vi "Register Events.vi"(0 "Display State In":T2={"WebView2 Ref"=refnum, "event callback refnum"=refnum, "Events"={"Navigation Complete Event"=refnum, "Source Changed Event"=refnum, "Document Title Changed Event"=refnum, "Status Bar Text Changed"=refnum, "Web Message Received"=refnum, "Window Close Requested"=refnum, "DOM Loaded"=refnum}, "Paths"={"Webview2 Native"=path "C:/Users/kleins/Desktop/webview2/microsoft.web.webview2.1.0.1370.28/build/native", "Edge Application"=path "", "User Data"=path ""}, "Environment Options"={"additionalBrowserArguments"="", "language"="", "targetCompatibleBrowserVersion"="", "allowSingleSignOnUsingOSPrimaryAccount"=FALSE}}, 9 "Container State":T5, 11 "error in (no error)":errorcluster) -> (4 "Display State Out":T2={"WebView2 Ref"=refnum, "event callback refnum"=refnum, "Events"={"Navigation Complete Event"=refnum, "Source Changed Event"=refnum, "Document Title Changed Event"=refnum, "Status Bar Text Changed"=refnum, "Web Message Received"=refnum, "Window Close Requested"=refnum, "DOM Loaded"=refnum}, "Paths"={"Webview2 Native"=path "C:/Users/kleins/Desktop/webview2/microsoft.web.webview2.1.0.1370.28/build/native", "Edge Application"=path "", "User Data"=path ""}, "Environment Options"={"additionalBrowserArguments"="", "language"="", "targetCompatibleBrowserVersion"="", "allowSingleSignOnUsingOSPrimaryAccount"=FALSE}}, 6 "Events":T1, 15 "error out":errorcluster)   [LabVIEW 2020, in "WebView2 Control.xctl"]
uses:
  WebView2 Control.xctl
  <vilib>/_xctls/Container State.ctl
  State.ctl
  E:/Labview/LV 2020/Libs/WebView2/LV-WebView2/Source/microsoft.web.webview2/lib/net45/Microsoft.Web.WebView2.WinForms.dll
  microsoft.web.webview2/lib/net45/Microsoft.Web.WebView2.WinForms.dll
  Events.ctl
  Paths.ctl
  Core Env Options.ctl
  _Raise Nav Complete Event.vi
  _Raise Navigation Starting Event.vi
  _Raise Source Changed Event.vi
  _Raise Document Title Changed.vi
  _Raise StatusBarTextChanged.vi
  _Raise WebMessageReceived.vi
  _Raise WindowCloseRequested.vi
  _Raise Dom Content Loaded.vi
  E:/Labview/LV 2020/Libs/WebView2/LV-WebView2/Source/microsoft.web.webview2/lib/net45/Microsoft.Web.WebView2.Core.dll
  microsoft.web.webview2/lib/net45/Microsoft.Web.WebView2.Core.dll
  <vilib>/_xctls/XControlSupport.lvlib
panel:
  # "Add Controls & Indicators that form the parameters of the method here. Hook them to the connector pane. Do not delete the controls & indicators that are already hooked to the connector pane.\n \nTo setup the parameters  for this method, right click on this item in the Project Tree & select \"Configure Method...\"."
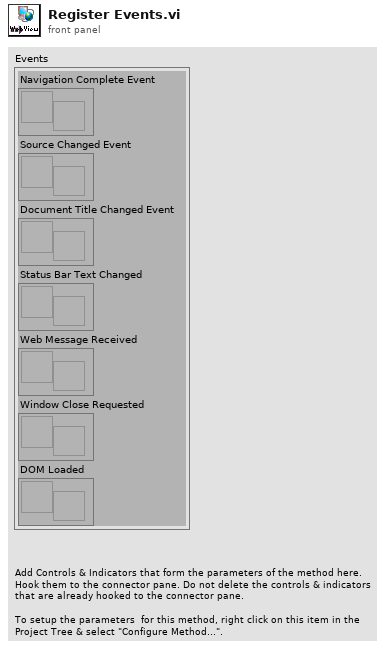
[diagram p1: front panel]
types:
  T1 = typedef "WebView2 Control.xctl/Events.ctl" = cluster{"Navigation Complete Event":refnum<user-event>, "Source Changed Event":refnum<user-event>, "Document Title Changed Event":refnum<user-event>, "Status Bar Text Changed":refnum<user-event>, "Web Message Received":refnum<user-event>, "Window Close Requested":refnum<user-event>, "DOM Loaded":refnum<user-event>}
  T2 = typedef "WebView2 Control.xctl/State.ctl" = cluster{"WebView2 Ref":refnum<data-value>, "event callback refnum":refnum<k27>, "Events":T1, "Paths":T3, "Environment Options":T4}
  T3 = typedef "WebView2 Control.xctl/Paths.ctl" = cluster{"Webview2 Native":path, "Edge Application":path, "User Data":path}
  T4 = typedef "WebView2 Control.xctl/Core Env Options.ctl" = cluster{"additionalBrowserArguments":string, "language":string, "targetCompatibleBrowserVersion":string, "allowSingleSignOnUsingOSPrimaryAccount":bool}
  T5 = typedef "XControlSupport.lvlib/Container State.ctl" = cluster{"Indicator?":bool, "Run Mode?":bool, " Refnum":refnum<vi>}
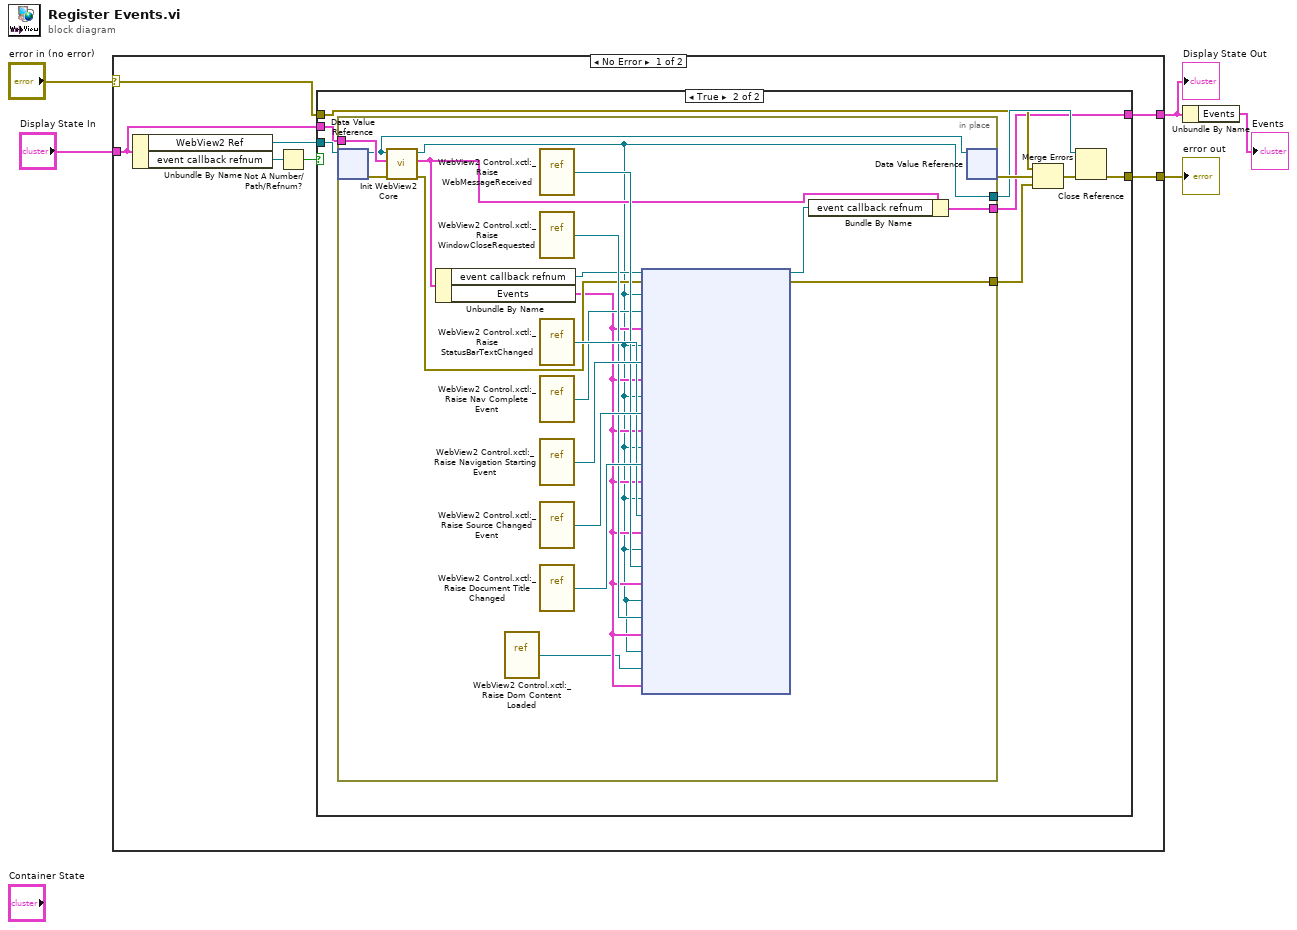
[diagram p0: block diagram]
diagram:
  n1 = case shown="No Error" "error in (no error)" {
    selector: "error in (no error)" -> [w9 w44]
    tunnel: [w8 w43] -> w2
    tunnel: "Display State In" -> [w11 w43]
    tunnel: [w10 w44] -> w4
    frame No Error {
      n2 = Unbundle By Name(w11) -> ("WebView2 Ref"=w12:refnum<data-value>, "event callback refnum"=w7:refnum<k27>)
      n3 = Not A Number/Path/Refnum?(number/path/refnum=w7) -> (NaN/Path/Refnum?=w6:bool)
      n4 = case shown="True" w6 {
        tunnel: w12 -> [_ w23]
        tunnel: w11 -> [w14 w22]
        tunnel: [w13 w21] -> w10
        tunnel: w9 -> [w13 w16]
        tunnel: [w14 w15] -> w8
        frame False {
        }
        frame True {
          n5 = in-place {
            in-place-border: [w42] -> w19
            in-place-border: [w24] -> w17
            in-place-border: w22 -> [w33]
            in-place-border: [w27] -> w15
            n6 = in-place-dvr #1(w23) -> (w32:refnum<k24>, w31:errorcluster)
            n7 = call "Init WebView2 Core.vi"("error in (no error)"=w31, "Display State In"=w33, "WebView In"=w32) -> ("error out"=w34:errorcluster, "Display State In 2"=w30:T2, "CoreWebView Out"=w24:refnum<k24>)  [unwired: 6 in]
            n8 = Unbundle By Name(w30) -> ("event callback refnum"=w29:refnum<k27>, "Events"=w26:T1)
            n9 = vi-ref "WebView2 Control.xctl:_Raise Dom Content Loaded.vi"() -> ("vi reference"=w25:refnum<vi>)
            n10 = vi-ref "WebView2 Control.xctl:_Raise WebMessageReceived.vi"() -> ("vi reference"=w37:refnum<vi>)
            n11 = vi-ref "WebView2 Control.xctl:_Raise WindowCloseRequested.vi"() -> ("vi reference"=w36:refnum<vi>)
            n12 = vi-ref "WebView2 Control.xctl:_Raise StatusBarTextChanged.vi"() -> ("vi reference"=w38:refnum<vi>)
            n13 = vi-ref "WebView2 Control.xctl:_Raise Nav Complete Event.vi"() -> ("vi reference"=w35:refnum<vi>)
            n14 = vi-ref "WebView2 Control.xctl:_Raise Navigation Starting Event.vi"() -> ("vi reference"=w41:refnum<vi>)
            n15 = vi-ref "WebView2 Control.xctl:_Raise Source Changed Event.vi"() -> ("vi reference"=w40:refnum<vi>)
            n16 = vi-ref "WebView2 Control.xctl:_Raise Document Title Changed.vi"() -> ("vi reference"=w39:refnum<vi>)
            n17 = node(w29, w34, w24, w35, w26, w24, w41, w26, w24, w40, w26, w24, w39, w26, w24, w38, w26, w24, w37, w26, w24, w36, w26, w24, w25, w26) -> (w28:refnum<k27>, w42:errorcluster)
            n18 = Bundle By Name(cluster=w30, "event callback refnum"=w28) -> (w27:T2)
            n19 = in-place-dvr #1(w32) -> (w20:errorcluster)  [unwired: 1 out]
          }
          n20 = Merge Errors(w16, w20, w19) -> (w18:errorcluster)
          n21 = Close Reference(reference=w17, error in (no error)=w18) -> (error out=w21:errorcluster)
        }
      }
    }
    frame Error {
    }
  }
  "Display State Out" <- w2
  "error out" <- w4
  n22 = Unbundle By Name(w2) -> ("Events"=→"Events":T1)
